vi "ALONE_IMAN.vi"(6 "Refresco(s)":dbl=0.01 caption="Elapsed Time (s)" format="%.3f", 8 "error in (no error)":errorcluster) -> (0 "Error Out":errorcluster, 7 "Enable":bool=TRUE)   [LabVIEW 2017]
uses:
  <vilib>/Analysis/baseanly.llb/Mean (DBL).vi
  cRIO_ZNB_AMI_GLOBALES.vi
  <vilib>/gmath/NI_Gmath.lvlib
  <vilib>/Analysis/NI_AALBase.lvlib
panel:
  in  "Gap":enum16{"gap 31mm", "gap 76 mm"}(ring)
  in  "Send":bool
  in  "q":i32=10 caption="Puntos, q" format="%#.0f"
  out "Array":dbl[](array[numeric])
  out "T Stable (T:yes)":bool caption="Stable"
  in  "sd max, %":dbl=100.0 caption="Desviacion max, %" format="%.2f"
  in  "Error max (T)":dbl=1.5 caption="Error" format="%.2f"
  out "Field Status":i32(ring) items=["MagnetUnknown"=0, "StablePersistent"=1, "WarmingSwitch"=2, "CoolingSwitch"=3, "StableDriven"=4, "Iterating"=5, "Charging"=6, "Discharging"=7, "CurrentError"=8, "MagnetFailure"=15]
  out "Num 1":i32
  out "Num 2":i32
  out "SetPoint(T).":dbl format="%.2f"
  in  "Setpoint B(T)":dbl format="%.2f"
  in  "Rate(T/min)":dbl=0.1 format="%.2f"
  out "CampoMagnet(T).":dbl format="%.2f"
  out "ERROR":bool
  out "Date":string caption="asd"
  out "Time":string
  in  "Refresh":bool
  in  "stop":bool
  # "Campo Magnetico (Aout0)"
  # "STATUS"
  # "SETTINGS"
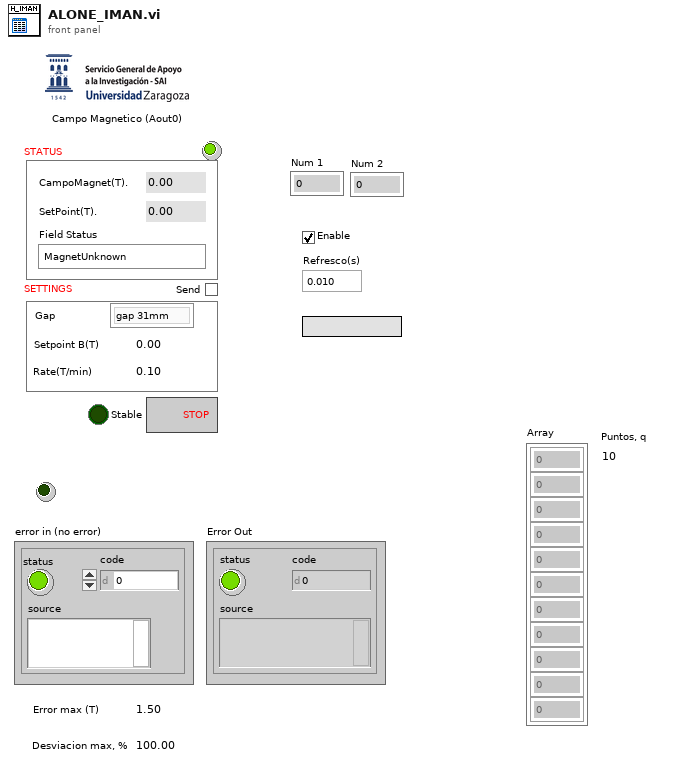
[diagram p1: front panel]
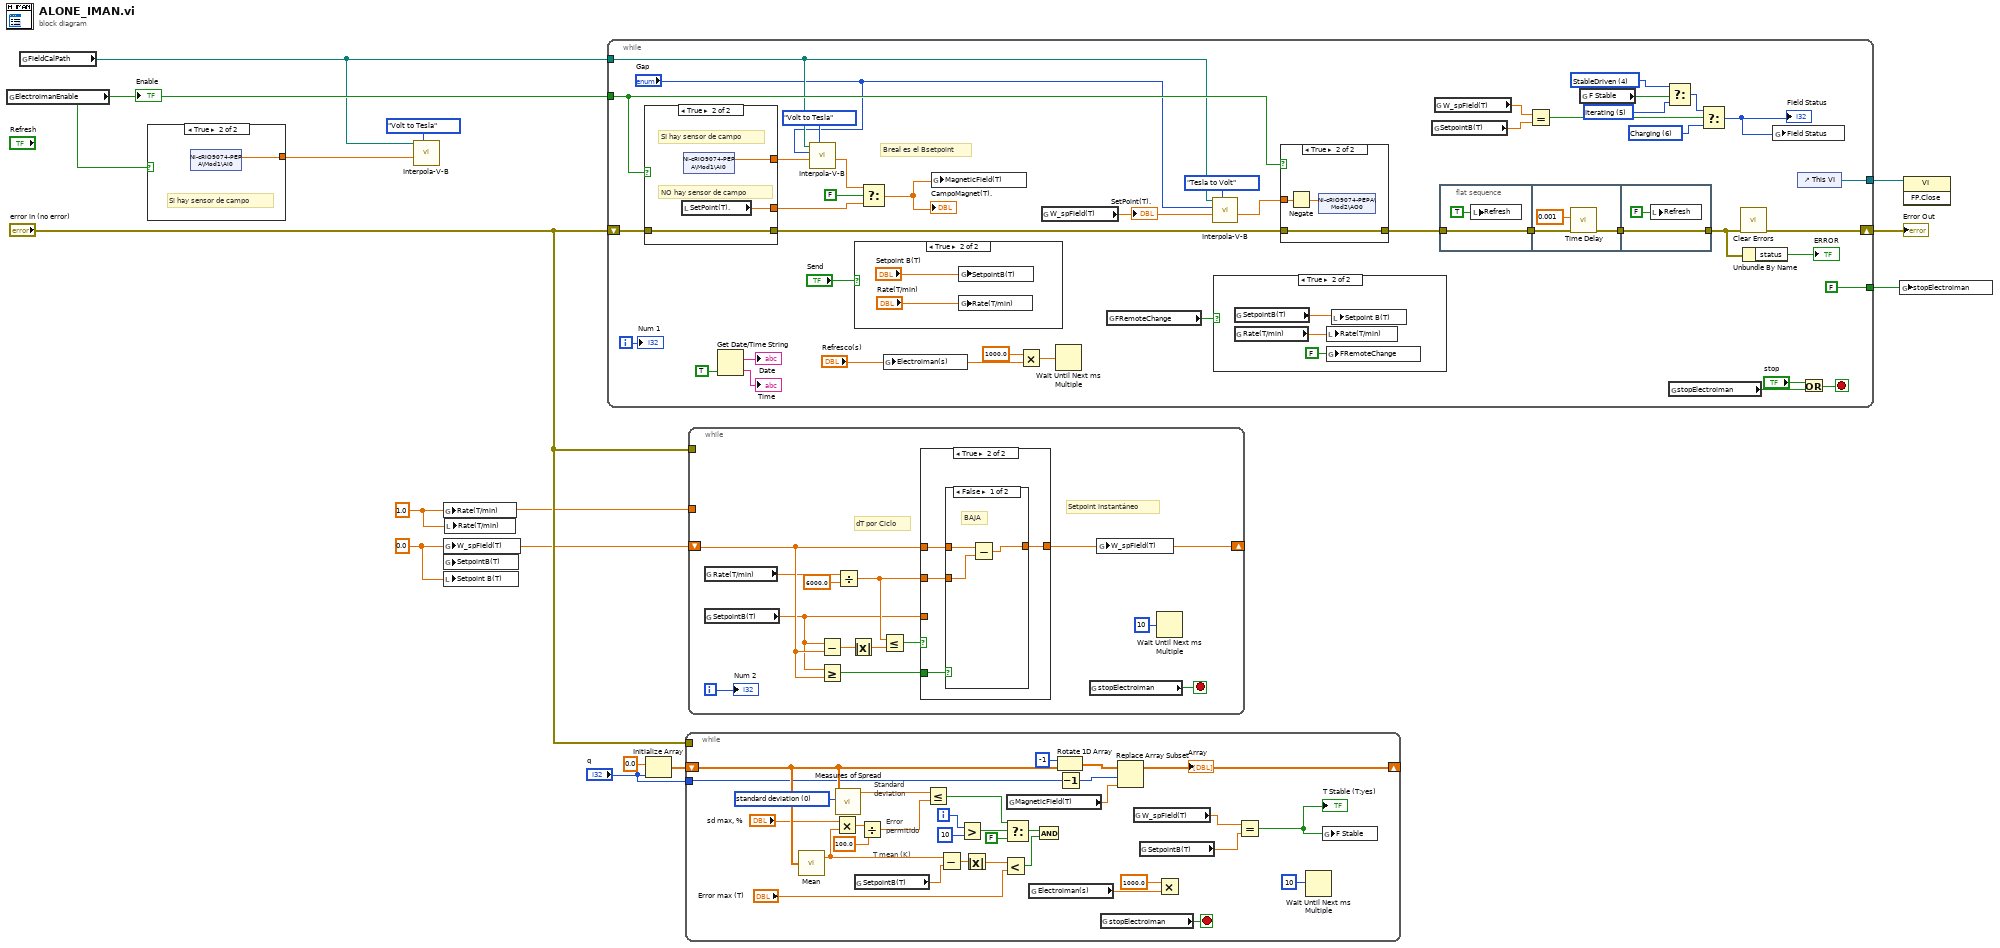
[diagram p0: block diagram]
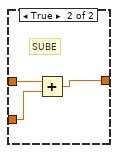
[diagram p3: hidden frame]
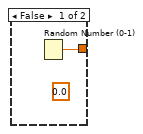
[diagram p4: hidden frame]
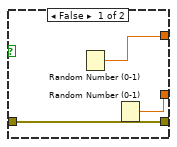
[diagram p8: hidden frame]
diagram:
  w4 = 0.0 ("W_spTemp(K)")
  w5 = 1.0 ("Rate(K/min)")
  n1 = global read "cRIO_ZNB_AMI_GLOBALES.vi" "ElectroimanEnable"() -> (w10:bool)
  "Enable" <- w10
  n2 = global read "cRIO_ZNB_AMI_GLOBALES.vi" "FieldCalPath"() -> (w1:path)
  n3 = case shown="True" w10 {
    tunnel: [w14 w15] -> w2
    frame False {
      (unwired) 0.0 ("W_spField(T)")
      n4 = Random Number (0-1)() -> (number: 0 to 1=w14:dbl)
    }
    frame True {
      # "Si hay sensor de campo"
      n5 = shared-variable "NI-cRIO9074-PEPA\\Mod1\\AI0"() -> (w15:dbl)  [unwired: 1 in, 1 out]
    }
  }
  n6 = call "Interpola-V-B.vi"("Modo"=enum16{"Volt to Tesla", "Tesla to Volt"}."Volt to Tesla", "INPUT"=w2, "FilePath"=w1) -> ()  [unwired: 7 in, 2 out]
  n7 = global write "cRIO_ZNB_AMI_GLOBALES.vi" "Rate(T/min)"(w5) -> ()
  n8 = global write "cRIO_ZNB_AMI_GLOBALES.vi" "W_spField(T)"(w4) -> ()
  n9 = global write "cRIO_ZNB_AMI_GLOBALES.vi" "SetpointB(T)"(w4) -> ()
  n10 = local write "Setpoint B(T)"(w4) -> ()
  n11 = local write "Rate(T/min)"(w5) -> ()
  n12 = while {
    shift-right: [w47] -> w11
    shift-left: "error in (no error)" -> [w40]
    tunnel: [FALSE ("stop")] -> w12
    tunnel: [w52] -> w13
    tunnel: w10 -> [w42]
    tunnel: w1 -> [w23]
    i -> [w43]
    stop <- w56 stop-if-true
    w29 = 6 items=["MagnetUnknown"=0, "StablePersistent"=1, "WarmingSwitch"=2, "CoolingSwitch"=3, "StableDriven"=4, "Iterating"=5, "Charging"=6, "Discharging"=7, "CurrentError"=8, "MagnetFailure"=15] ("Field Status")
    w31 = 5 items=["MagnetUnknown"=0, "StablePersistent"=1, "WarmingSwitch"=2, "CoolingSwitch"=3, "StableDriven"=4, "Iterating"=5, "Charging"=6, "Discharging"=7, "CurrentError"=8, "MagnetFailure"=15] ("Field Status")
    w30 = 4 items=["MagnetUnknown"=0, "StablePersistent"=1, "WarmingSwitch"=2, "CoolingSwitch"=3, "StableDriven"=4, "Iterating"=5, "Charging"=6, "Discharging"=7, "CurrentError"=8, "MagnetFailure"=15] ("Field Status")
    # "Breal es el Bsetpoint"
    n13 = case shown="True" w42 {
      tunnel: [w70 w72] -> w24
      tunnel: w40 -> [w69 w73]
      tunnel: [w69 w73] -> w41
      tunnel: [w68 w71] -> w19
      frame False {
        n14 = Random Number (0-1)() -> (number: 0 to 1=w70:dbl)
        n15 = Random Number (0-1)() -> (number: 0 to 1=w68:dbl)
      }
      frame True {
        # "NO hay sensor de campo"
        # "SI hay sensor de campo"
        n16 = local read "SetPoint(T)."() -> (w71:dbl)
        n17 = shared-variable "NI-cRIO9074-PEPA\\Mod1\\AI0"() -> (w72:dbl)  [unwired: 1 in, 1 out]
      }
    }
    n18 = Get Date/Time String(want seconds? (F)=TRUE) -> (date string=→"Date":string, time string=→"Time":string)  [unwired: 2 in]
    n19 = call "Interpola-V-B.vi"("Modo"=enum16{"Volt to Tesla", "Tesla to Volt"}."Volt to Tesla", "INPUT"=w24, "Gap"="Gap", "FilePath"=w23) -> ("OUTPUT"=w18:dbl)  [unwired: 6 in, 1 out]
    n20 = case shown="True" "Send" {
      frame False {
      }
      frame True {
        n21 = global write "cRIO_ZNB_AMI_GLOBALES.vi" "SetpointB(T)"("Setpoint B(T)") -> ()
        n22 = global write "cRIO_ZNB_AMI_GLOBALES.vi" "Rate(T/min)"("Rate(T/min)") -> ()
      }
    }
    n23 = Select(t=w18, s=FALSE, f=w19) -> (s? t:f=w17:dbl)
    "CampoMagnet(T)." <- w17
    n24 = global write "cRIO_ZNB_AMI_GLOBALES.vi" "Electroiman(s)"("Refresco(s)") -> ()
    n25 = global write "cRIO_ZNB_AMI_GLOBALES.vi" "MagneticField(T)"(w17) -> ()
    n26 = Multiply(x=1000.0, y="Refresco(s)") -> (x*y=w48:dbl)
    n27 = global read "cRIO_ZNB_AMI_GLOBALES.vi" "W_spField(T)"() -> (w22:dbl)
    "SetPoint(T)." <- w22
    n28 = Wait Until Next ms Multiple(millisecond multiple=w48) -> ()  [unwired: 1 out]
    n29 = global read "cRIO_ZNB_AMI_GLOBALES.vi" "FRemoteChange"() -> (w27:bool)
    n30 = call "Interpola-V-B.vi"("Modo"=enum16{"Volt to Tesla", "Tesla to Volt"}."Tesla to Volt", "INPUT"=w22, "Gap"="Gap", "FilePath"=w23) -> ("OUTPUT"=w21:dbl)  [unwired: 6 in, 1 out]
    n31 = case shown="True" w27 {
      frame False {
      }
      frame True {
        n32 = global read "cRIO_ZNB_AMI_GLOBALES.vi" "SetpointB(T)"() -> (w61:dbl)
        n33 = global read "cRIO_ZNB_AMI_GLOBALES.vi" "Rate(T/min)"() -> (w60:dbl)
        n34 = local write "Rate(T/min)"(w60) -> ()
        n35 = global write "cRIO_ZNB_AMI_GLOBALES.vi" "FRemoteChange"(FALSE ("TRemoteChange")) -> ()
        n36 = local write "Setpoint B(T)"(w61) -> ()
      }
    }
    n37 = case shown="True" w42 {
      tunnel: w21 -> [_ w66]
      tunnel: w41 -> [w64 w67]
      tunnel: [w64 w67] -> w39
      frame False {
      }
      frame True {
        n38 = Negate(x=w66) -> (-x=w65:dbl)
        n39 = shared-variable "NI-cRIO9074-PEPA\\Mod2\\AO0"(w65) -> ()  [unwired: 1 in, 1 out]
      }
    }
    n40 = global read "cRIO_ZNB_AMI_GLOBALES.vi" "SetpointB(T)"() -> (w35:dbl)
    n41 = global read "cRIO_ZNB_AMI_GLOBALES.vi" "W_spField(T)"() -> (w36:dbl)
    n42 = flat-sequence {
      tunnel: w39 -> [w74]
      tunnel: [w74] -> w46
      tunnel: w46 -> [w77]
      tunnel: [w76] -> w45
      tunnel: [w79] -> w44
      tunnel: w45 -> [w79]
      frame #0 {
        n43 = local write "Refresh"(TRUE ("Refresh")) -> ()
      }
      frame #1 {
        n44 = call "Time Delay"("error in (no error)"=w77, "Delay Time (s)"=0.001) -> ("error out"=w76:errorcluster)  [unwired: 9 in]
      }
      frame #2 {
        n45 = local write "Refresh"(FALSE ("Refresh")) -> ()
      }
    }
    n46 = Equal?(x=w36, y=w35) -> (x = y?=w34:bool)
    n47 = global read "cRIO_ZNB_AMI_GLOBALES.vi" "F Stable"() -> (w32:bool)
    n48 = Select(t=w30, s=w32, f=w31) -> (s? t:f=w33:i32)
    n49 = global read "cRIO_ZNB_AMI_GLOBALES.vi" "stopElectroiman"() -> (w51:bool)
    n50 = Select(t=w33, s=w34, f=w29) -> (s? t:f=w37:i32)
    "Field Status" <- w37
    n51 = call <vilib>:"Clear Errors.vi"("error in (no error)"=w44) -> ("error out"=w47:errorcluster)  [unwired: 5 in, 1 out]
    n52 = Unbundle By Name(w44) -> ("status"=→"ERROR":bool)
    n53 = global write "cRIO_ZNB_AMI_GLOBALES.vi" "Field Status"(w37) -> ()
    n54 = control-ref of="This VI"() -> (w52:refnum<vi>)
    n55 = Or(x="stop", y=w51) -> (x .or. y?=w56:bool)
    "Num 1" <- w43
  }
  "Error Out" <- w11
  n56 = Initialize Array(0.0 ("element"), "q") -> (w9:dbl[])
  n57 = while {
    tunnel: "q" -> [w93]
    shift-right: [w108] -> _
    shift-left: w9 -> [w94]
    tunnel: "error in (no error)" -> [_]
    i -> [w85]
    stop <- w112 stop-if-true
    w98 = 0 items=["standard deviation", "range", "mean absolute deviation", "interquartile range"] ("type")
    # "Error\npermitido"
    # "Standard\ndeviation"
    # "T mean (K)"
    n58 = call-poly <vilib>:"Mean.vi"("X"=w94) -> ("mean"=w91:dbl)  [unwired: 1 out]
    n59 = Multiply(x="sd max, %", y=w91) -> (x*y=w103:dbl)
    n60 = call <vilib>:"Measures of Spread.vi"("type"=w98, "x array"=w94) -> ("spread value"=w107:dbl)  [unwired: 8 in, 1 out]
    n61 = global read "cRIO_ZNB_AMI_GLOBALES.vi" "SetpointB(T)"() -> (w90:dbl)
    n62 = Divide(x=w103, y=100.0) -> (x/y=w102:dbl)
    n63 = Less Or Equal?(x=w107, y=w102) -> (x <= y?=w105:bool)
    n64 = Subtract(x=w91, y=w90) -> (x-y=w101:dbl)
    n65 = Greater?(x=w85, y=10) -> (0:w106:bool)
    n66 = Absolute Value(x=w101) -> (abs(x)=w100:dbl)
    n67 = Less?(x=w100, y="Error max (T)") -> (x < y?=w99:bool)
    n68 = Select(t=w105, s=w106, f=FALSE ("TdownStable (T:yes)")) -> (s? t:f=w104:bool)
    n69 = global read "cRIO_ZNB_AMI_GLOBALES.vi" "MagneticField(T)"() -> (w88:dbl)
    n70 = global read "cRIO_ZNB_AMI_GLOBALES.vi" "Electroiman(s)"() -> (w87:dbl)
    n71 = And(x=w104, y=w99) -> ()  [unwired: 1 out]
    n72 = Rotate 1D Array(1:w94, 2:-1 ("n")) -> (0:w110:dbl[])
    n73 = Decrement(x=w93) -> (x-1=w111:i32)
    n74 = global read "cRIO_ZNB_AMI_GLOBALES.vi" "stopElectroiman"() -> (w112:bool)
    n75 = Replace Array Subset(array=w110, new element=w88, index=w111) -> (w108:dbl[])
    "Array" <- w108
    n76 = global read "cRIO_ZNB_AMI_GLOBALES.vi" "W_spField(T)"() -> (w82:dbl)
    n77 = global read "cRIO_ZNB_AMI_GLOBALES.vi" "SetpointB(T)"() -> (w84:dbl)
    n78 = Multiply(x=1000.0, y=w87) -> ()  [unwired: 1 out]
    n79 = Equal?(x=w82, y=w84) -> (x = y?=w83:bool)
    "T Stable (T:yes)" <- w83
    n80 = Wait Until Next ms Multiple(millisecond multiple=i64 10 ("Period")) -> ()  [unwired: 1 out]
    n81 = global write "cRIO_ZNB_AMI_GLOBALES.vi" "F Stable"(w83) -> ()
  }
  n82 = while {
    shift-right: [w118] -> _
    shift-left: w4 -> [w123]
    tunnel: "error in (no error)" -> [_]
    tunnel: w5 -> [_]
    i -> [w114]
    stop <- w115 stop-if-true
    # "Setpoint instantáneo"
    # "dT por Ciclo"
    n83 = global read "cRIO_ZNB_AMI_GLOBALES.vi" "Rate(T/min)"() -> (w117:dbl)
    n84 = global read "cRIO_ZNB_AMI_GLOBALES.vi" "SetpointB(T)"() -> (w116:dbl)
    n85 = Subtract(x=w116, y=w123) -> (x-y=w122:dbl)
    n86 = Greater Or Equal?(x=w116, y=w123) -> (x >= y?=w125:bool)
    n87 = Divide(x=w117, y=6000.0) -> (x/y=w121:dbl)
    n88 = Absolute Value(x=w122) -> (abs(x)=w120:dbl)
    n89 = Less Or Equal?(x=w121, y=w120) -> (x <= y?=w119:bool)
    n90 = case shown="True" w119 {
      tunnel: w116 -> [w126 _]
      tunnel: w121 -> [_ w127]
      tunnel: w123 -> [_ w130]
      tunnel: [w126 w129] -> w118
      tunnel: w125 -> [_ w128]
      frame False {
      }
      frame True {
        n91 = case shown="False" w128 {
          tunnel: w130 -> [w132 w135]
          tunnel: [w133 w136] -> w129
          tunnel: w127 -> [w131 w134]
          frame False {
            # "BAJA"
            n92 = Subtract(x=w132, y=w131) -> (x-y=w133:dbl)
          }
          frame True {
            # "SUBE"
            n93 = Add(x=w135, y=w134) -> (x+y=w136:dbl)
          }
        }
      }
    }
    n94 = global read "cRIO_ZNB_AMI_GLOBALES.vi" "stopElectroiman"() -> (w115:bool)
    n95 = global write "cRIO_ZNB_AMI_GLOBALES.vi" "W_spField(T)"(w118) -> ()
    n96 = Wait Until Next ms Multiple(millisecond multiple=i64 10 ("Period")) -> ()  [unwired: 1 out]
    "Num 2" <- w114
  }
  n97 = global write "cRIO_ZNB_AMI_GLOBALES.vi" "stopElectroiman"(w12) -> ()
  n98 = invoke class="VI" method="FP.Close"(reference=w13) -> ()  [unwired: 2 in, 3 out]
